vi "Disconnect from stage.vi"(8 "error in (no error)":errorcluster, 10 "Hardware State":T1) -> (0 "error out":errorcluster, 2 "Hardware State Out":T1)   [LabVIEW 2015, in "XYZStage.lvlib"]
uses:
  XYZStage.lvlib
  XYZStage State.ctl
  XYZStage Loop State.ctl
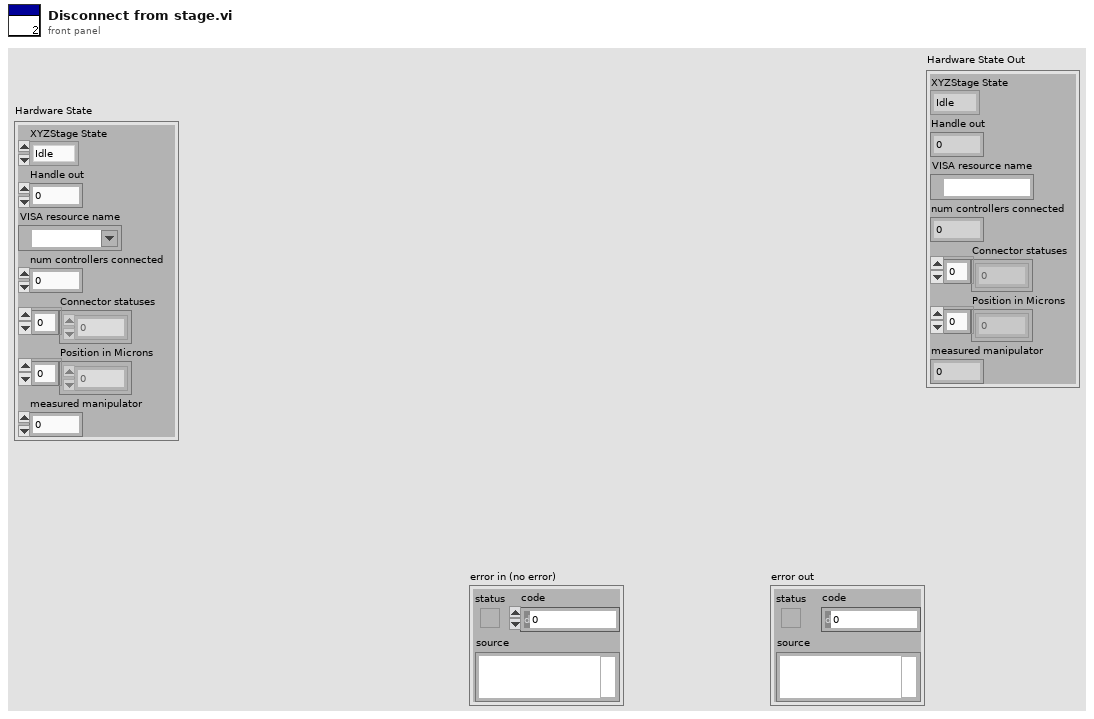
[diagram p1: front panel]
types:
  T1 = typedef "XYZStage.lvlib/XYZStage State.ctl" = cluster{"XYZStage State":T2, "Handle out":u32, "VISA resource name":refnum<visa-resource-name>, "num controllers connected":u8, "Connector statuses":u8[], "Position in Microns":dbl[], "measured manipulator":u8}
  T2 = typedef "XYZStage.lvlib/XYZStage Loop State.ctl" = enum16{"Idle", "Connected", "Moving"}
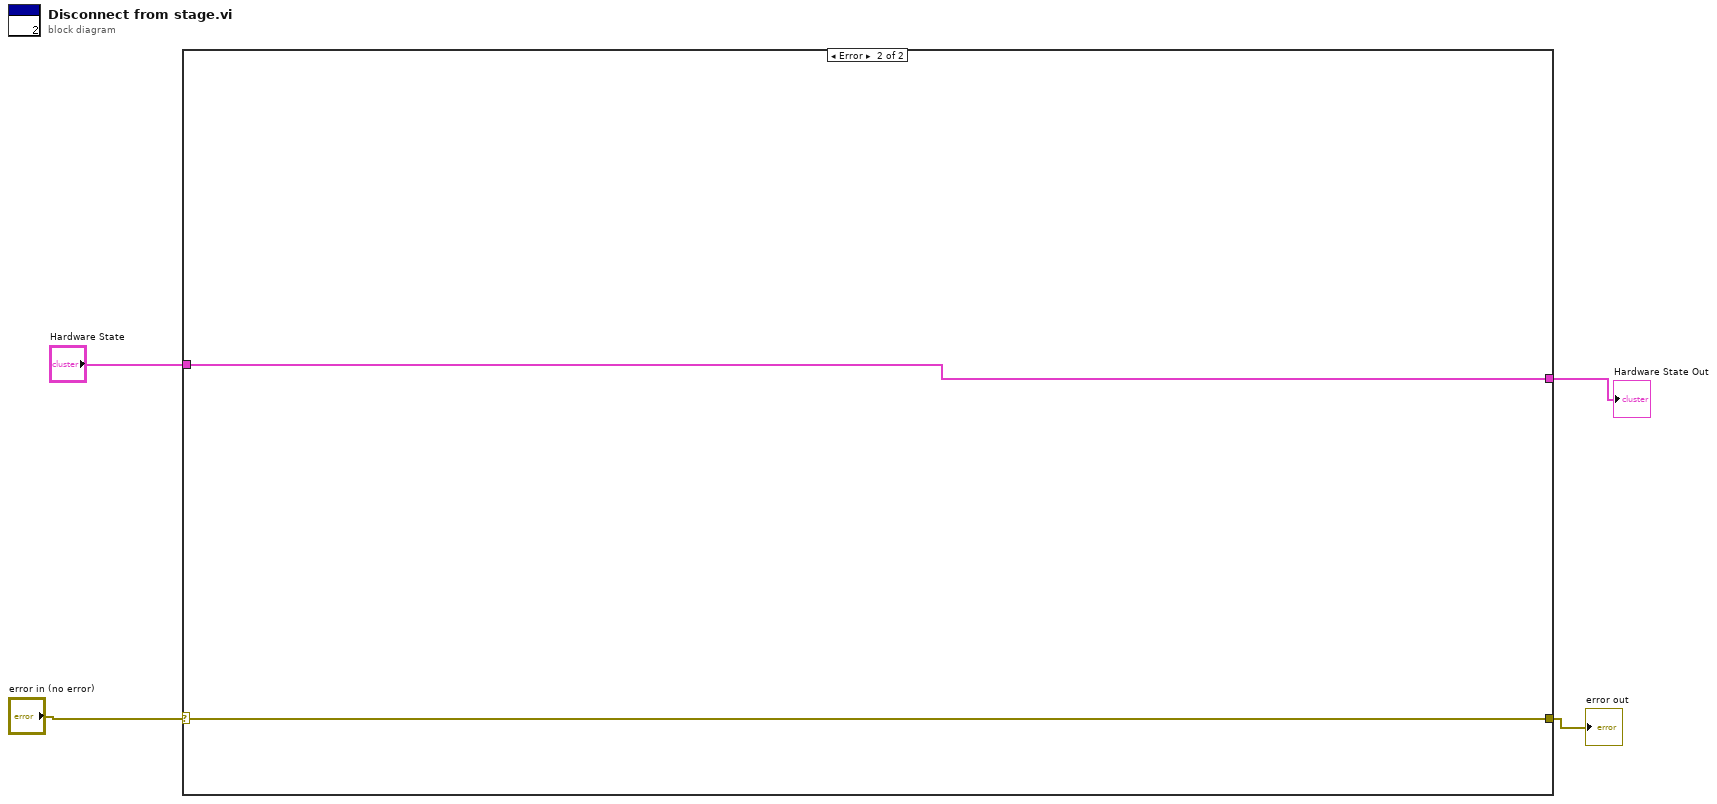
[diagram p0: block diagram]
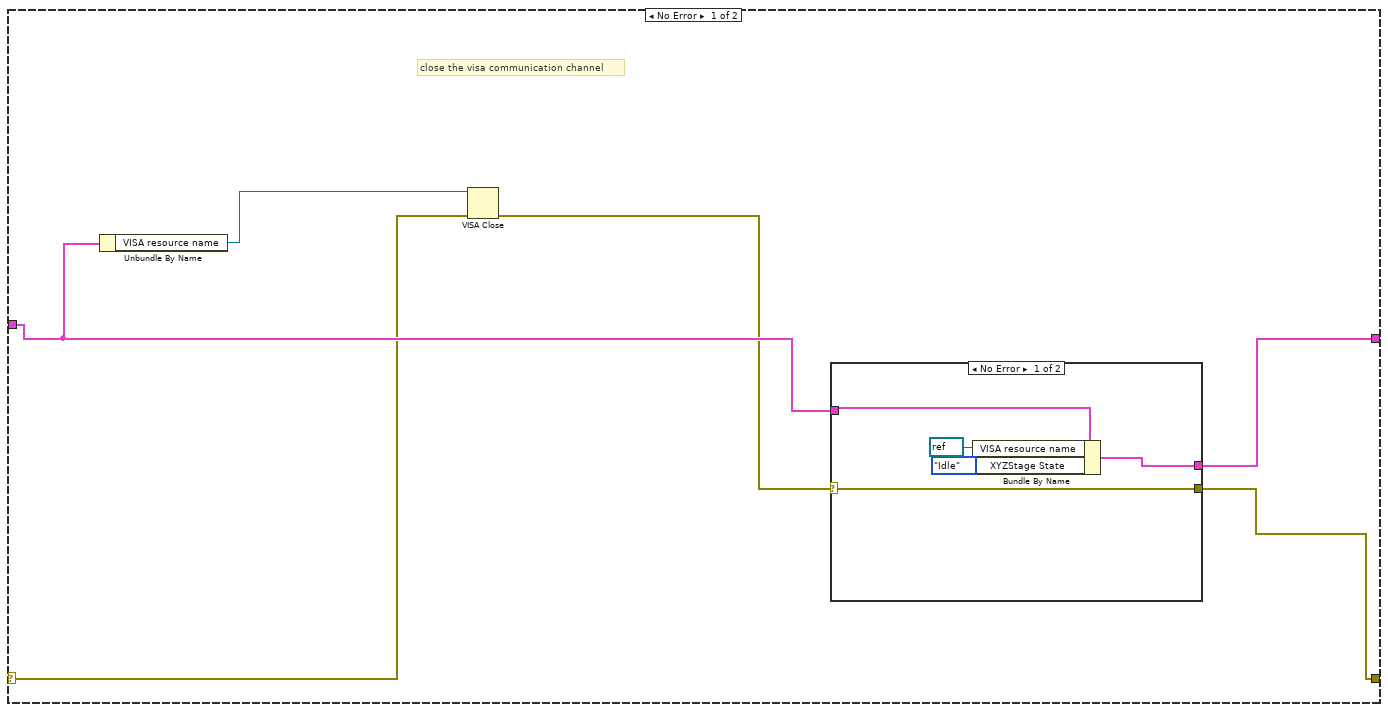
[diagram p2: hidden frame]
diagram:
  n1 = case shown="Error" "error in (no error)" {
    selector: "error in (no error)" -> [w6 w19]
    tunnel: [w9 w19] -> w3
    tunnel: [w10 w18] -> w2
    tunnel: "Hardware State" -> [w8 w18]
    frame No Error {
      # "close the visa communication channel"
      n2 = Unbundle By Name(w8) -> ("VISA resource name"=w7:refnum<visa-resource-name>)
      n3 = VISA Close(VISA resource name=w7, error in (no error)=w6) -> (error out=w5:errorcluster)
      n4 = case shown="No Error" w5 {
        selector: w5 -> [w12 w16]
        tunnel: w8 -> [w15 w17]
        tunnel: [w14 w17] -> w10
        tunnel: [w12 w16] -> w9
        frame No Error {
          n5 = Bundle By Name(cluster=w15, "VISA resource name"=refnum<visa-resource-name> refnum, "XYZStage State"=XYZStage_Loop_State."Idle") -> (w14:T1)
        }
        frame Error {
        }
      }
    }
    frame Error {
    }
  }
  "error out" <- w3
  "Hardware State Out" <- w2
